vi "ReadChannel.vi"(5 "Channel":i32, 6 "error in":errorcluster) -> (0 "error out":errorcluster, 4 "Value":bool)   [LabVIEW 2014]
doc: "Read the current value of the specified channel.\n\nThe channel must be configured as an input before calling this VI."
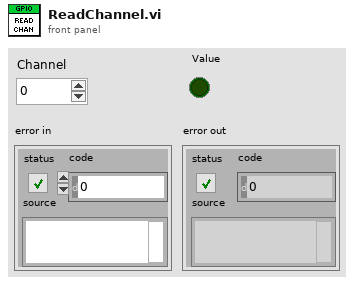
[diagram p1: front panel]
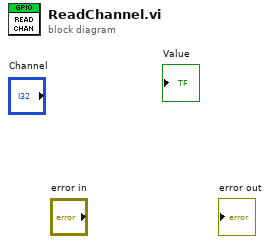
[diagram p0: block diagram]
diagram:
